vi "Configure Trigger (Pattern).vi"(6 "Duration High Threshold (3E-8 S)":dbl=3e-08, 7 "Duration Low Threshold (2E-8 S)":dbl=2e-08, 8 "error in (no error)":errorcluster, 9 "Qualifier (0: Entered)":i32(ring) items=["Entered", "Greater Than", "Less Than", "Within Range", "Outside Range", "Timeout"], 10 "Pattern Value (XXXXXXXXXXXXXXXXXXXX)":string="XXXXXXXXXXXXXXXXXXXX", 11 "VISA resource name":refnum<visa-resource-name>) -> (0 "error out":errorcluster, 3 "VISA resource name out":refnum<visa-resource-name>)   [LabVIEW 2015, in "Agilent 2000 3000 X-Series.lvlib"]
doc: "Configures the pattern trigger mode."
uses:
  Agilent 2000 3000 X-Series.lvlib
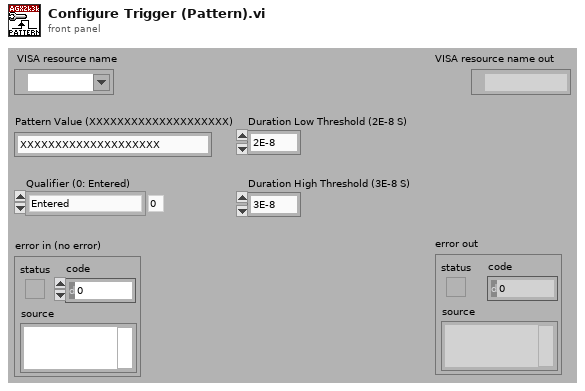
[diagram p1: front panel]
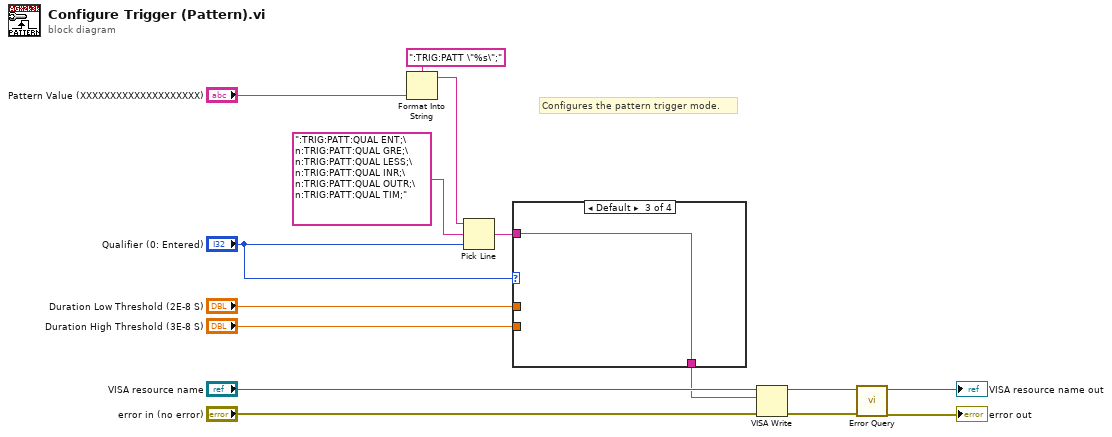
[diagram p0: block diagram]
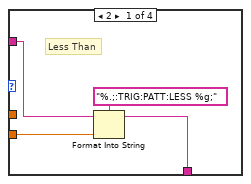
[diagram p2: hidden frame]
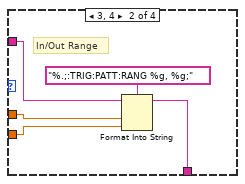
[diagram p3: hidden frame]
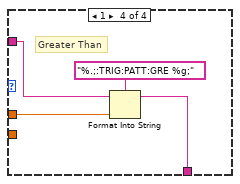
[diagram p4: hidden frame]
diagram:
  # "Configures the pattern trigger mode."
  n1 = Format Into String(format string=":TRIG:PATT \"%s\";", "Pattern Value (XXXXXXXXXXXXXXXXXXXX)") -> (resulting string=w3:string)  [unwired: 2 in, 1 out]
  n2 = Pick Line(string ("")=w3, multi-line string=":TRIG:PATT:QUAL ENT;\n:TRIG:PATT:QUAL GRE;\n:TRIG:PATT:QUAL LESS;\n:TRIG:PATT:QUAL INR;\n:TRIG:PATT:QUAL OUTR;\n:TRIG:PATT:QUAL TIM;", line index="Qualifier (0: Entered)") -> (output string=w2:string)
  n3 = case shown="Default" "Qualifier (0: Entered)" {
    tunnel: "Duration Low Threshold (2E-8 S)" -> [_ w23 _ w29]
    tunnel: "Duration High Threshold (3E-8 S)" -> [w18 w22 _ _]
    tunnel: w2 -> [w17 w21 w25 w27]
    tunnel: [w16 w20 w25 w26] -> w1
    frame 2 {
      # "Less Than"
      n4 = Format Into String(format string="%.;:TRIG:PATT:LESS %g;", initial string=w17, w18) -> (resulting string=w16:string)  [unwired: 1 in, 1 out]
    }
    frame 3, 4 {
      # "In/Out Range"
      n5 = Format Into String(format string="%.;:TRIG:PATT:RANG %g, %g;", initial string=w21, w23, w22) -> (resulting string=w20:string)  [unwired: 1 in, 1 out]
    }
    frame Default {
    }
    frame 1 {
      # "Greater Than"
      n6 = Format Into String(format string="%.;:TRIG:PATT:GRE %g;", initial string=w27, w29) -> (resulting string=w26:string)  [unwired: 1 in, 1 out]
    }
  }
  n7 = VISA Write(VISA resource name="VISA resource name", write buffer=w1, error in (no error)="error in (no error)") -> (VISA resource name out=w10:refnum<visa-resource-name>, error out=w9:errorcluster)  [unwired: 1 out]
  n8 = call "Error Query.vi"("error in (no error)"=w9, "VISA resource name"=w10) -> ("error out"=→"error out":errorcluster, "VISA resource name out"=→"VISA resource name out":refnum<visa-resource-name>)  [unwired: 8 out]
